vi "Calculate Prime Number using MathScript Node 2012 NIVerified .vi"() -> ()   [LabVIEW 2012]
doc: "Demonstrates how to calculate 1001st prime number using Math Script."
uses:
  <vilib>/imath/engines/lvmath2/RunTimeEngine/ErrorHandling/NIMS_Finalize Error.vi
  <vilib>/imath/engines/lvmath2/RunTimeEngine/Managers/WorkSpace/UID Generator.vi
  <vilib>/imath/engines/lvmath2/RunTimeEngine/Managers/SymbolTable/Clear UID.vi
  <vilib>/imath/engines/lvmath2/RunTimeEngine/NodeEndStatement/NIMS_NodeEndStatement_Output.vi
  <instcachedir>/0/NIMS_NodeEndStatement_Output_53EC0D466D134D7ABD903AC30B43404B.lvgen/NIMS_NodeEndStatement_Output_53EC0D466D134D7ABD903AC30B43404B_012.vi
  <vilib>/imath/engines/lvmath2/RunTimeEngine/BuiltInFunctions/is_prime/NIMS_is_prime.vi
  <vilib>/imath/engines/lvmath2/RunTimeEngine/RunTimeType/NIMS_RunTimeType_From StrictType (excl LVString).vi
  <instcachedir>/0/NIMS_RunTimeType_From StrictType (excl LVString)_AC52D965D0864706932D20A05968E122.lvgen/NIMS_RunTimeType_From StrictType (excl LVString)_AC52D965D0864706932D20A05968E122_000.vi
  <vilib>/imath/engines/lvmath2/RunTimeEngine/RunTimeType/NIMS_RunTimeType_Set Source Original Bool.vi
  <vilib>/imathl/engines/lvmath/Functions/Error Handling/Create Error.vi
  <vilib>/imath/engines/lvmath2/RunTimeEngine/LocalVariableDefStatement/MC_LocalVariableDefStatement_Display.vi
  <vilib>/imath/engines/lvmath2/RunTimeEngine/Managers/SymbolTable/NIMS_WorkSpace.lvlib
panel:
  out "1001st Prime Number":dbl
  # "Overview: Demonstrates how to calculate 1001st prime number using MathScript Node.\nRequirements: LabVIEW 2012 (or compatible), Math Script RT module\nInstructions:\n1. Run the program\n2. The program takes a few seconds to compute the first 1001 prime numbers\n3. The 1001st prime number will be displayed"
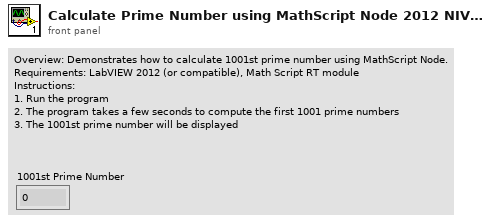
[diagram p1: front panel]
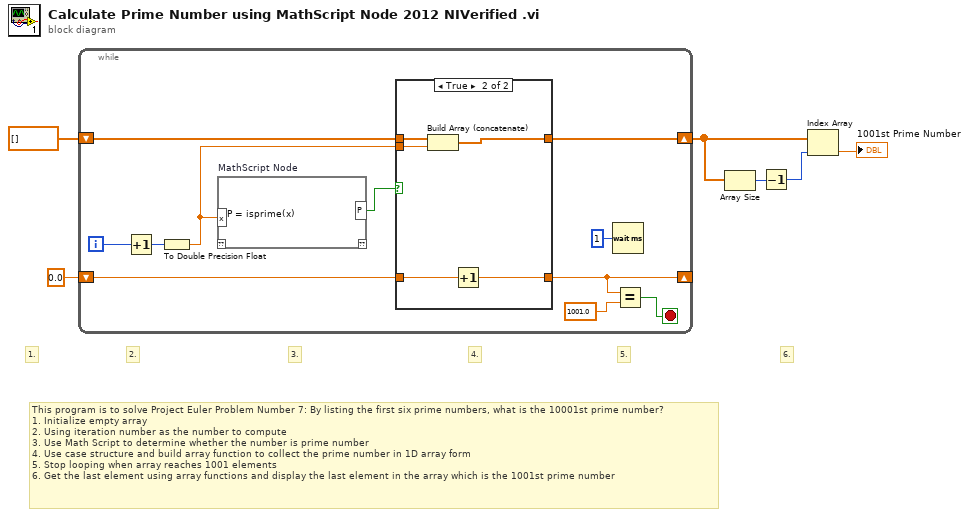
[diagram p0: block diagram]
diagram:
  # "6."
  # "5."
  # "4."
  # "3."
  # "2."
  # "1."
  # "This program is to solve Project Euler Problem Number 7: By listing the first six prime numbers, what is the 10001st prime number?\n1. Initialize empty array\n2. Using iteration number as the number to compute\n3. Use Math Script to determine whether the number is prime number\n4. Use case structure and build array function to collect the prime number in 1D array form\n5. Stop looping when array reaches 1001 elements\n6. Get the last element using array functions and display the last element in the array which is the 1001st prime number"
  n1 = while {
    shift-right: [w12] -> w2
    shift-left: dbl[] [] -> [w15]
    shift-right: [w8] -> _
    shift-left: 0.0 -> [w11]
    i -> [w17]
    stop <- w10 stop-if-true
    n2 = Increment(x=w17) -> (x+1=w16:i32)
    n3 = To Double Precision Float(number=w16) -> (double precision float=w14:dbl)
    n4 = mathscript code="P = isprime(x)"("x"=w14) -> ("P"=w13:bool)  [unwired: 1 in, 1 out]
    n5 = case shown="True" w13 {
      tunnel: w15 -> [w19 w24]
      tunnel: w14 -> [_ w23]
      tunnel: [w19 w22] -> w12
      tunnel: w11 -> [w18 w21]
      tunnel: [w18 w20] -> w8
      frame False {
      }
      frame True {
        n6 = Build Array (concatenate) "Build Array"(w24, w23) -> (w22:dbl[])
        n7 = Increment(x=w21) -> (x+1=w20:dbl)
      }
    }
    n8 = Wait (ms)(milliseconds to wait=u32 1) -> ()  [unwired: 1 out]
    n9 = Equal?(x=w8, y=1001.0) -> (x = y?=w10:bool)
  }
  n10 = Array Size(array=w2) -> (size(s)=w4:i32)
  n11 = Decrement(x=w4) -> (x-1=w3:i32)
  n12 = Index Array "Index Array"(array=w2, index=w3) -> (element=→"1001st Prime Number":dbl)
